vi "Auto Setup Core.vi"(8 "error in (no error)":errorcluster, 11 "CS++Scope":refnum<class "CS++Scope.lvclass">) -> (0 "error out":errorcluster, 3 "CS++Scope out":refnum<class "CS++Scope.lvclass">)   [LabVIEW 2014, in "CS++Scope.lvlib" / "CS++Scope.lvclass"]
doc: "This VI automatically configures the instrument.\n\nNotes:\n\nNote \n(1) When you call this VI, the oscilloscope senses the input signal and automatically configures many of the instrument settings. The settings no longer match the cache values for the corresponding properties. Therefore, this VI invalidates all property cache values.\n\n(2) This VI is part of the IviScopeAutoSetup [AS] extension group."
uses:
  CS++Scope.lvclass
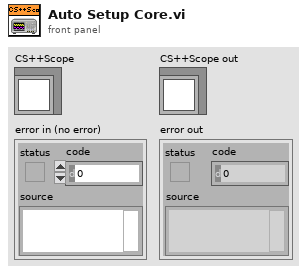
[diagram p1: front panel]
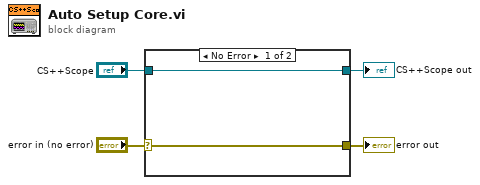
[diagram p0: block diagram]
diagram:
  n1 = case shown="No Error" "error in (no error)" {
    selector: "error in (no error)" -> [w5 w8]
    tunnel: [w5 w8] -> w3
    tunnel: [w6 w7] -> w2
    tunnel: "CS++Scope" -> [w6 w7]
    frame No Error {
    }
    frame Error {
    }
  }
  "error out" <- w3
  "CS++Scope out" <- w2
